vi "Gif.DataSubBlocks.vi"(0 "data":string, 9 "offset":i32, 11 "error in (no error)":errorcluster) -> (4 "data out":string, 6 "SubBlock values":string[](array[string]), 10 "offset out":i32, 15 "error out":errorcluster)   [LabVIEW 2019]
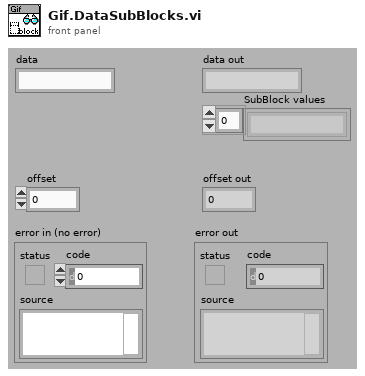
[diagram p1: front panel]
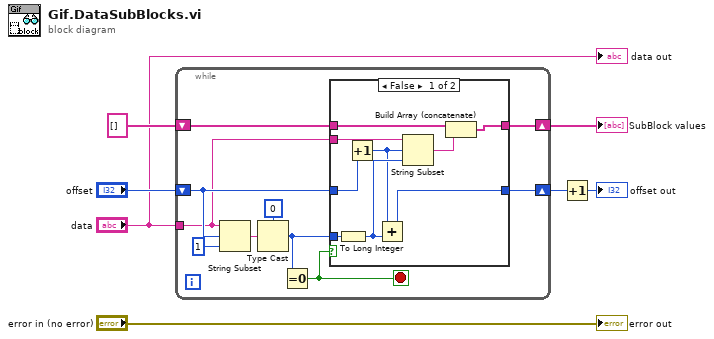
[diagram p0: block diagram]
diagram:
  n1 = while {
    tunnel: "data" -> [w10]
    shift-right: [w11] -> w5
    shift-left: "offset" -> [w12]
    shift-right: [w9] -> w2
    shift-left: string[] [] -> [w8]
    stop <- w14 stop-if-true
    n2 = String Subset(string=w10, offset (0)=w12, length (rest)=1 ("length (rest)")) -> (substring=w16:string)
    n3 = Type Cast(type=u8 0 ("element"), x=w16) -> (*(type *) &x=w13:u8)
    n4 = Equal To 0?(x=w13) -> (x = 0?=w14:bool)
    n5 = case shown="False" w14 {
      tunnel: w13 -> [w26 _]
      tunnel: w12 -> [w23 w28]
      tunnel: [w25 w28] -> w11
      tunnel: w10 -> [w24 _]
      tunnel: [w18 w27] -> w9
      tunnel: w8 -> [w20 w27]
      frame False {
        n6 = To Long Integer(number=w26) -> (32bit integer=w22:i32)
        n7 = Increment(x=w23) -> (x+1=w21:i32)
        n8 = Add(x=w21, y=w22) -> (x+y=w25:i32)
        n9 = String Subset(string=w24, offset (0)=w21, length (rest)=w22) -> (substring=w19:string)
        n10 = Build Array (concatenate)(w20, w19) -> (w18:string[])
      }
      frame True {
      }
    }
  }
  "SubBlock values" <- w2
  n11 = Increment(x=w5) -> (x+1=→"offset out":i32)
  "data out" <- "data"
  "error out" <- "error in (no error)"
